vi "PH_StatusHandler.get Status.vi"(0 "VI in":refnum<vi>, 5 "error in":errorcluster) -> (14 "VI out":refnum<vi>, 16 "Status":T1 items=["no info", "off/false/out", "on/true/in", "Failure", "Alarm", "Status 1", "Status 2", "Status 3"], 19 "error out":errorcluster)   [LabVIEW 2014, in "PH_StatusHandler.lvlib"]
uses:
  PH_StatusHandler.lvlib
  PH_StatusHandler.Status.ctl
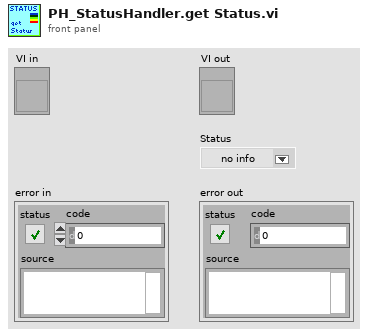
[diagram p1: front panel]
types:
  T1 = typedef "PH_StatusHandler.lvlib/PH_StatusHandler.Status.ctl" = i16
  T2 = typedef "PH_StatusHandler.lvlib/PH_StatusHandler.i attribute.ctl" = cluster{"GUI Ref":refnum<vi>, "Value":T1, "Service ID":i32}
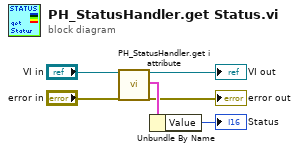
[diagram p0: block diagram]
diagram:
  n1 = call "PH_StatusHandler.get i attribute.vi"("i ref in"="VI in", "error in (no error)"="error in") -> ("i ref out"=→"VI out":refnum<vi>, "i attribute"=w5:T2, "error out"=→"error out":errorcluster)  [unwired: 15 in]
  n2 = Unbundle By Name(w5) -> ("Value"=→"Status":T1)
